vi "LVPortProcessMatlabPropertyUpdates.vi"(8 "error in":errorcluster, 11 "pID":string) -> (0 "error out":errorcluster)   [LabVIEW 2017]
uses:
  Properties/LVPortControlBindingInfoType.ctl
  Properties/LVPortControlBindingDirectionEnum.ctl
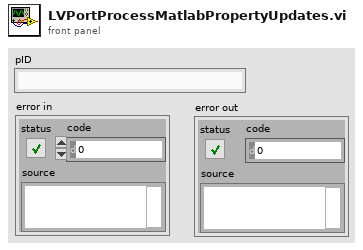
[diagram p1: front panel]
types:
  T1 = typedef "LVPortControlBindingDirectionEnum.ctl" = enum16{"BiDirectional", "ToMatlab", "ToLabview"}
  T2 = typedef "LVPortControlBindingInfoType.ctl" = cluster{"Bound Control":refnum<vi>, "Name":string, "Direction":T1, "Event Register":refnum<event-registration>}
  T3 = typedef "Dictionary Object RefNum__ogtk.ctl" = refnum<k1>
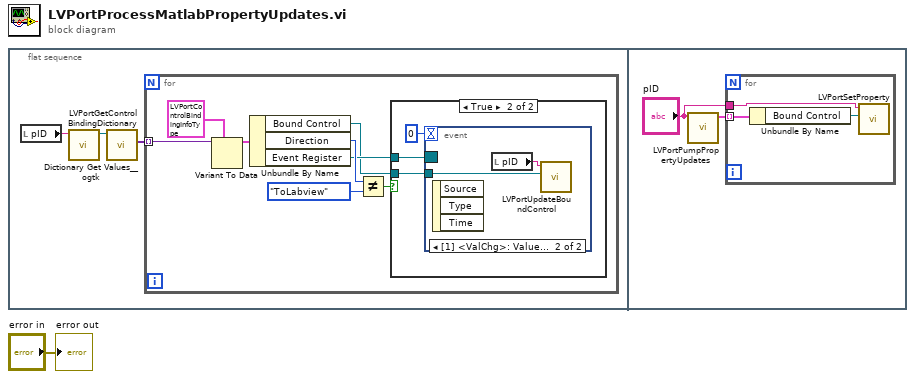
[diagram p0: block diagram]
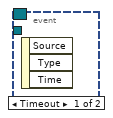
[diagram p3: hidden frame]
diagram:
  n1 = flat-sequence {
    frame #0 {
      n2 = local read "pID"() -> (w4:string)
      n3 = call "LVPortGetControlBindingDictionary.vi"("pID"=w4) -> ("Refnum out"=w3:T3)  [unwired: 10 in]
      n4 = call <userlib>:"Dictionary Get Values__ogtk.vi"("dictionary"=w3) -> ("values"=w2:variant[])  [unwired: 8 in, 2 out]
      n5 = for {
        tunnel: w2 -> [w12] mode=indexing
        n6 = Variant To Data(type=T2 {"Bound Control"=refnum, "Name"="", "Direction"=enum."BiDirectional", "Event Register"=refnum} ("Control Binding Info"), Variant=w12) -> (data=w10:T2)  [unwired: 1 in, 1 out]
        n7 = Unbundle By Name(w10) -> ("Bound Control"=w5:refnum<vi>, "Direction"=w9:T1, "Event Register"=w6:refnum<event-registration>)
        n8 = Not Equal?(x=w9, y=LVPortControlBindingDirectionEnum."ToLabview") -> (x != y?=w7:bool)
        n9 = case shown="True" w7 {
          tunnel: w6 -> [_ w15]
          tunnel: w5 -> [_ w14]
          frame False {
          }
          frame True {
            n10 = event shown="[1] <ValChg>: Value Change" {
              selector: w15 -> [_ _]
              dyn-events: _ -> [_ _]
              timeout: 0 -> [_ _]
              tunnel: w14 -> [_ w17]
              event Timeout {
                n11 = event-data() -> ()  [unwired: 1 in, 3 out]
              }
              event Value Change {
                n12 = event-data() -> ()  [unwired: 1 in, 3 out]
                n13 = local read "pID"() -> (w16:string)
                n14 = call "LVPortUpdateBoundControl.vi"("Control To Update"=w17, "pID"=w16) -> ()  [unwired: 9 in, 1 out]
              }
            }
          }
        }
      }
    }
    frame #1 {
      n15 = call "LVPortPumpPropertyUpdates.vi"("pID"="pID") -> ("Updating Bound Control Infos"=w19:T2[])  [unwired: 10 in]
      n16 = for {
        tunnel: w19 -> [w21] mode=indexing
        tunnel: "pID" -> [w22]
        n17 = Unbundle By Name(w21) -> ("Bound Control"=w20:refnum<vi>)
        n18 = call "LVPortSetProperty.vi"("Value"=w20, "pID"=w22) -> ()  [unwired: 8 in, 2 out]
      }
    }
  }
  "error out" <- "error in"
